vi "ErrorMngmt_Write.vi"(8 "error in (no error)":errorcluster, 11 "Queue in":refnum<queue>) -> (0 "error out":errorcluster, 3 "Queue out":refnum<queue>)   [LabVIEW 2015]
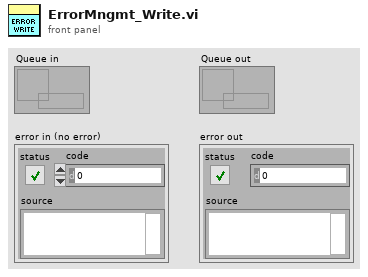
[diagram p1: front panel]
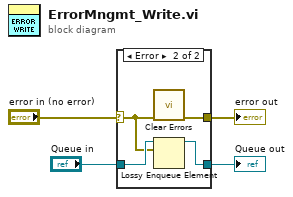
[diagram p0: block diagram]
diagram:
  n1 = case shown="Error" "error in (no error)" {
    selector: "error in (no error)" -> [w5 w9]
    tunnel: "Queue in" -> [w6 w10]
    tunnel: [w5 w8] -> w3
    tunnel: [w6 w7] -> w4
    frame No Error {
    }
    frame Error {
      n2 = call <vilib>:"Clear Errors.vi"("error in (no error)"=w9) -> ("error out"=w8:errorcluster)  [unwired: 5 in, 1 out]
      n3 = Lossy Enqueue Element(queue=w10, element=w9) -> (queue out=w7:refnum<queue>)  [unwired: 1 in, 3 out]
    }
  }
  "error out" <- w3
  "Queue out" <- w4
